vi "InitDataConPane.vi"(7 "VI Reference":refnum<vi>, 8 "error in (no error)":errorcluster) -> (0 "error out":errorcluster)   [LabVIEW 2009, in "HGF_VisitorGenerator.lvlib"]
doc: "link conPane of visitors appendData2Variant.vi"
uses:
  HGF_VisitorGenerator.lvlib
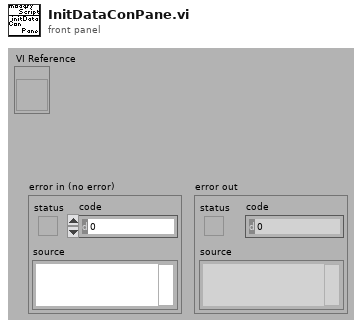
[diagram p1: front panel]
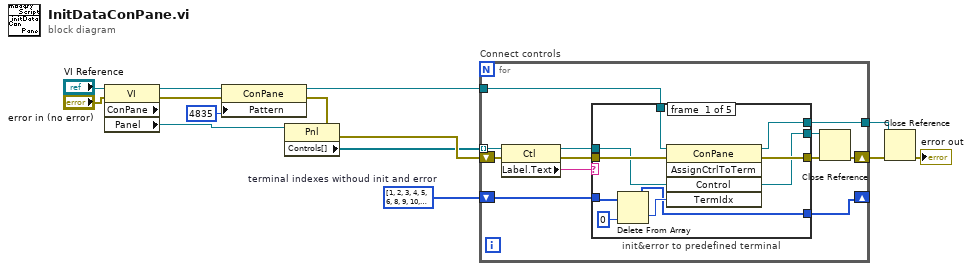
[diagram p0: block diagram]
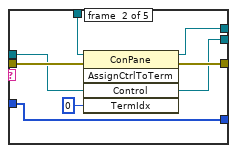
[diagram p2: hidden frame]
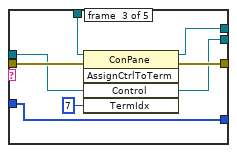
[diagram p3: hidden frame]
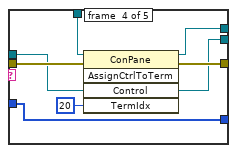
[diagram p4: hidden frame]
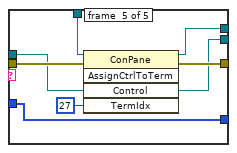
[diagram p5: hidden frame]
diagram:
  w1 = u32[] [1, 2, 3, 4, 5, 6, 8, 9, 10, 11, 12, 13, 14, 15, 16, 17, 18, 19, 21, 22, 23, 24, 25, 26]  # terminal indexes withoud init and error
  n1 = property class="VI"(reference="VI Reference", error in="error in (no error)") -> (error out=w6:errorcluster, "ConPane"=w7:refnum<vi>, "Panel"=w11:refnum<vi>)  [unwired: 1 out]
  n2 = property class="ConPane"(reference=w7, error in=w6, "Pattern"=u32 4835) -> (reference out=w4:refnum<vi>, error out=w5:errorcluster)
  n3 = property class="Pnl"(reference=w11, error in=w5) -> (error out=w12:errorcluster, "Controls[]"=w9:refnum<vi>[])  [unwired: 1 out]
  n4 = for "Connect controls" {
    shift-right: [w19] -> w2
    shift-left: w12 -> [w26]
    tunnel: w9 -> [w25] mode=indexing
    tunnel: w4 -> [w22]
    tunnel: [w21] -> w3
    shift-right: [w15] -> _
    shift-left: w1 -> [w16]
    n5 = property class="Ctl"(reference=w25, error in=w26) -> (reference out=w23:refnum<vi>, error out=w20:errorcluster, "Label.Text"=w24:string)
    n6 = case "init&error to predefined terminal" shown="\"error out\"" w24 {
      tunnel: w23 -> [w31 w38 w45 w52 w59]
      tunnel: w22 -> [w35 w42 w49 w56 w63]
      tunnel: [w34 w41 w48 w55 w62] -> w21
      tunnel: w20 -> [w33 w40 w47 w54 w61]
      tunnel: [w32 w39 w46 w53 w60] -> w18
      tunnel: [w31 w38 w45 w52 w59] -> w17
      tunnel: w16 -> [w30 w37 w44 w51 w58]
      tunnel: [w27 w37 w44 w51 w58] -> w15
      frame #0 {
        n7 = Delete From Array(array=w30, index=0) -> (deleted portion=w28:u32, array with subset deleted=w27:u32[])  [unwired: 1 in]
        n8 = invoke class="ConPane" method="AssignCtrlToTerm"(reference=w35, error in=w33, "Control"=w31, "TermIdx"=w28) -> (reference out=w34:refnum<vi>, error out=w32:errorcluster)  [unwired: 1 in, 3 out]
      }
      frame #1 {
        n9 = invoke class="ConPane" method="AssignCtrlToTerm"(reference=w42, error in=w40, "Control"=w38, "TermIdx"=u32 0 ("Terminal Index")) -> (reference out=w41:refnum<vi>, error out=w39:errorcluster)  [unwired: 1 in, 3 out]
      }
      frame #2 {
        n10 = invoke class="ConPane" method="AssignCtrlToTerm"(reference=w49, error in=w47, "Control"=w45, "TermIdx"=u32 7 ("Terminal Index")) -> (reference out=w48:refnum<vi>, error out=w46:errorcluster)  [unwired: 1 in, 3 out]
      }
      frame #3 {
        n11 = invoke class="ConPane" method="AssignCtrlToTerm"(reference=w56, error in=w54, "Control"=w52, "TermIdx"=u32 20 ("Terminal Index")) -> (reference out=w55:refnum<vi>, error out=w53:errorcluster)  [unwired: 1 in, 3 out]
      }
      frame #4 {
        n12 = invoke class="ConPane" method="AssignCtrlToTerm"(reference=w63, error in=w61, "Control"=w59, "TermIdx"=u32 27 ("Terminal Index")) -> (reference out=w62:refnum<vi>, error out=w60:errorcluster)  [unwired: 1 in, 3 out]
      }
    }
    n13 = Close Reference(reference=w17, error in (no error)=w18) -> (error out=w19:errorcluster)
  }
  n14 = Close Reference(reference=w3, error in (no error)=w2) -> (error out=→"error out":errorcluster)
